vi "Pre Launch Init.vi"(11 "File Actor in":refnum<class "File Actor.lvclass">) -> (0 "error out":errorcluster, 3 "File Actor out":refnum<class "File Actor.lvclass">)   [LabVIEW 2014, in "File Library.lvlib" / "File Actor.lvclass"]
doc: "Retrieve file related information from the configuration file and open a new file."
uses:
  File Actor.lvclass
  reusable/Command/Command.lvclass
  reusable/Session APIs/Session Log/System Log.lvclass
  reusable/Session APIs/Session Log/System Log.lvclass/System Log.ctl
  reusable/Session APIs/File Access/Config Data/Config Data.lvclass
  reusable/Session APIs/File Access/Config Data/Config Data.lvclass/Config Data.ctl
  File Actor.lvclass/File Actor.ctl
  reusable/Session APIs/Session Log/Accessors/Write Main Path.vi
  reusable/Session APIs/File Access/Config Data/Accessors/Write Cfg Path.vi
  Controller/xGlobal Data.vi
  SuperActor/Ex Nested.lvclass
  <userlib>/_Session Fwk/Session - Root.lvclass
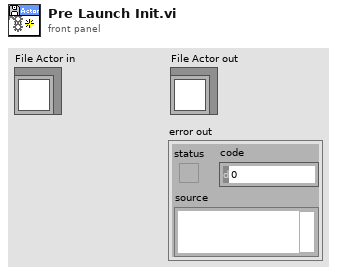
[diagram p1: front panel]
types:
  T1 = typedef "Session - Root.lvclass/Session Handle.ctl" = refnum<data-value>
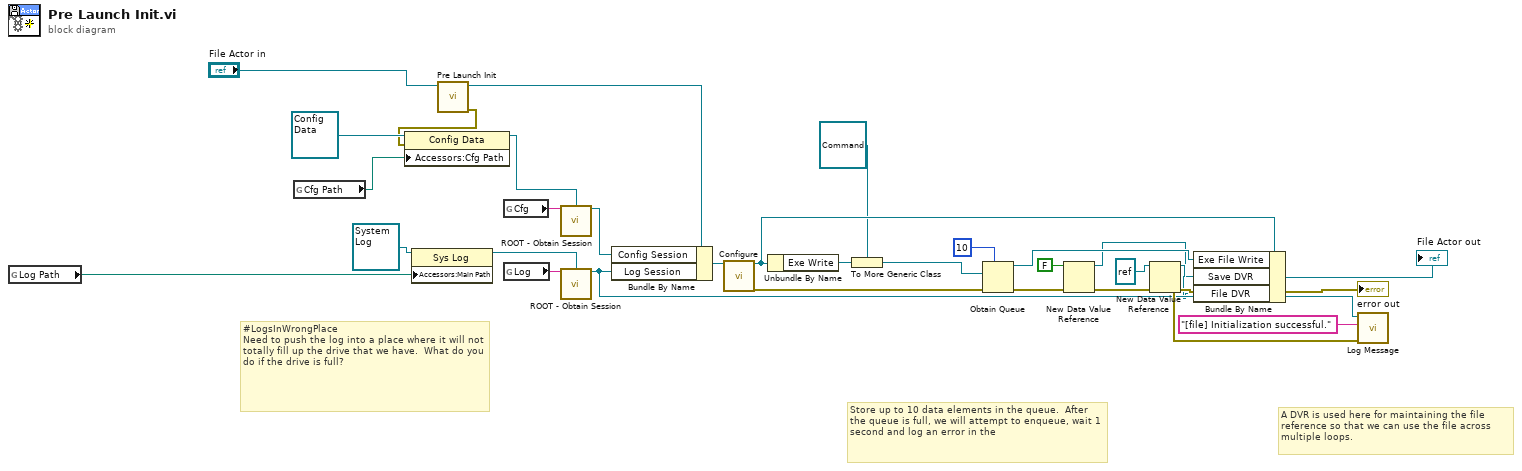
[diagram p0: block diagram]
diagram:
  # "#LogsInWrongPlace\nNeed to push the log into a place where it will not totally fill up the drive that we have.  What do you do if the drive is full?"
  # "Store up to 10 data elements in the queue.  After the queue is full, we will attempt to enqueue, wait 1 second and log an error in the"
  # "A DVR is used here for maintaining the file reference so that we can use the file across multiple loops."
  n1 = global read "xGlobal Data.vi" "Log Path"() -> (w13:path)
  n2 = global read "xGlobal Data.vi" "Cfg Path"() -> (w7:path)
  n3 = property class="Sys Log"(reference=refnum<class "System Log.lvclass"> refnum ("Sys Log"), "Accessors:Main Path"=w13) -> (reference out=w12:refnum<class "System Log.lvclass">)  [unwired: 1 in, 1 out]
  n4 = call-parent "Pre Launch Init.vi"("Ex Nested in"="File Actor in") -> ("error out"=w1:errorcluster, "Ex Nested out"=w2:refnum<class "File Actor.lvclass">)  [unwired: 9 in]
  n5 = property class="Config Data"(reference=refnum<class "Config Data.lvclass"> refnum ("Config Data"), error in=w1, "Accessors:Cfg Path"=w7) -> (reference out=w6:refnum<class "Config Data.lvclass">)  [unwired: 1 out]
  n6 = global read "xGlobal Data.vi" "Cfg"() -> (w15:string)
  n7 = global read "xGlobal Data.vi" "Log"() -> (w16:string)
  n8 = call <userlib>:"ROOT - Obtain Session.vi"("Session Name ()"=w15, "OBJ - Session"=w6) -> ("Session Handle"=w10:T1)  [unwired: 11 in, 2 out]
  n9 = call <userlib>:"ROOT - Obtain Session.vi"("Session Name ()"=w16, "OBJ - Session"=w12) -> ("Session Handle"=w9:T1)  [unwired: 11 in, 2 out]
  n10 = Bundle By Name(cluster=w2, "Config Session"=w10, "Log Session"=w9) -> (w11:refnum<class "File Actor.lvclass">)
  n11 = call "Configure.vi"("File Actor in"=w11) -> ("File Actor out"=w26:refnum<class "File Actor.lvclass">, "error out"=w20:errorcluster)  [unwired: 17 in]
  n12 = Unbundle By Name(w26) -> ("Exe Write"=w24:refnum<class "Exe Write.lvclass">)
  n13 = To More Generic Class(target class=refnum<class "Command.lvclass"> refnum ("CMD"), reference=w24) -> (generic class reference=w22:refnum<class "Command.lvclass">)
  n14 = Obtain Queue(max queue size (-1, unlimited)=10, element data type=w22, error in (no error)=w20) -> (queue out=w21:refnum<queue>, error out=w18:errorcluster)  [unwired: 2 in, 1 out]
  n15 = New Data Value Reference(data value=FALSE, error in=w18) -> (data value reference=w4:refnum<data-value>, error out=w17:errorcluster)
  n16 = New Data Value Reference(data value=refnum<file> refnum ("File Ref"), error in=w17) -> (data value reference=w5:refnum<data-value>, error out=w27:errorcluster)
  "error out" <- w27
  n17 = Bundle By Name(cluster=w26, "Exe File Write"=w21, "Save DVR"=w4, "File DVR"=w5) -> (→"File Actor out":refnum<class "File Actor.lvclass">)
  n18 = call "Log Message.vi"("error in"=w27, "MSG In"="[file] Initialization successful.", "session in"=w9) -> ()  [unwired: 7 in, 2 out]
